vi "多参数数据插入.vi"(8 "error in (no error)":errorcluster caption="错误输入（无错误）", 9 "编号":string, 10 "columns enable":T1, 11 "data in":T2) -> (0 "error out":errorcluster)   [LabVIEW 2016, in "斯坦道多参数.lvlib"]
uses:
  <vilib>/Utility/sysdir.llb/System Directory Type.ctl
  <vilib>/addons/database/Auxilliary.llb/DB Tools Parameter Info.ctl
  <vilib>/addons/database/Auxilliary.llb/DB Tools DataTypes.ctl
  <vilib>/addons/database/Auxilliary.llb/DB Tools Parameter Dir.ctl
  <vilib>/addons/database/Auxilliary.llb/DB Tools Column Info.ctl
  <vilib>/addons/database/Auxilliary.llb/DB Tools Format Datetime String (Time Stamp).vi
  <vilib>/addons/database/Connection.llb/DB Tools Open Connec (String).vi
  <vilib>/addons/database/Connection.llb/Conn Execute.vi
  <vilib>/addons/database/Recordset.llb/Rec Destroy - Connection.vi
  <vilib>/addons/database/Command.llb/Cmd Set Parameter Value (C).vi
  <vilib>/addons/database/Command.llb/Cmd Execute.vi
  <vilib>/addons/database/Recordset.llb/Rec Destroy - Command.vi
  <vilib>/addons/database/Command.llb/Cmd Delete.vi
  <vilib>/addons/database/NI_Database_API.lvlib
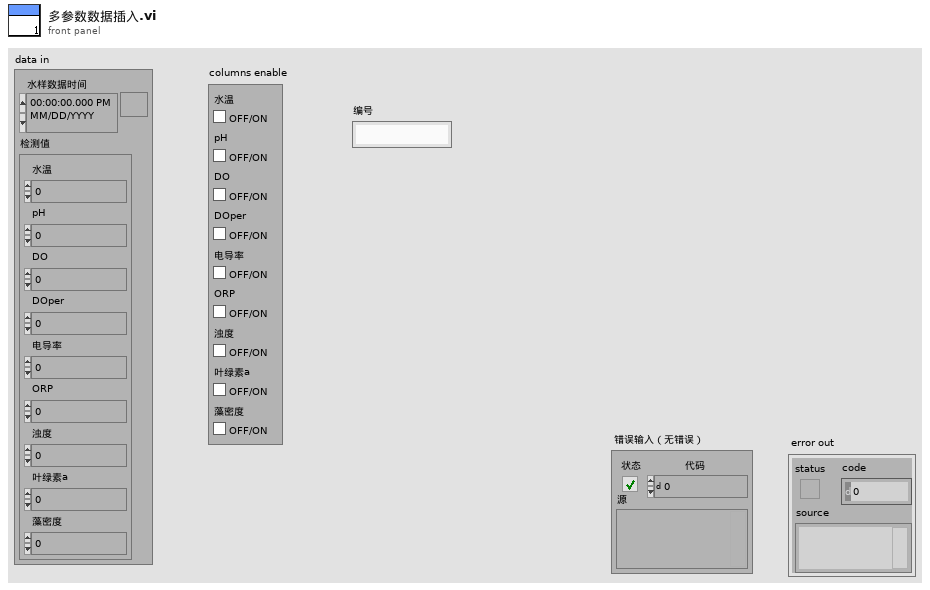
[diagram p1: front panel]
types:
  T1 = cluster{"水温":bool, "pH":bool, "DO":bool, "DOper":bool, "电导率":bool, "ORP":bool, "浊度":bool, "叶绿素a":bool, "藻密度":bool}
  T2 = cluster{"水样数据时间":timestamp, "检测值":cluster{"水温":dbl, "pH":dbl, "DO":dbl, "DOper":dbl, "电导率":dbl, "ORP":dbl, "浊度":dbl, "叶绿素a":dbl, "藻密度":dbl}}
  T3 = typedef "System Directory Type.ctl" = i32
  T4 = cluster{"水温":dbl, "pH":dbl, "DO":dbl, "DOper":dbl, "电导率":dbl, "ORP":dbl, "浊度":dbl, "叶绿素a":dbl, "藻密度":dbl}
  T5 = typedef "NI_Database_API.lvlib/DB Tools Column Info.ctl" = cluster{"column name":string, "data type":T6, "size":i32, "allow null?":bool}
  T6 = typedef "NI_Database_API.lvlib/DB Tools DataTypes.ctl" = enum16{"String", "Long (I32)", "Single (SGL)", "Double (DBL)", "Date/Time", "Binary"}
  T7 = typedef "NI_Database_API.lvlib/DB Tools Parameter Info.ctl" = cluster{"parameter name":string, "type":T6, "direction":T8, "value":variant}
  T8 = typedef "NI_Database_API.lvlib/DB Tools Parameter Dir.ctl" = enum32{"Input", "Output", "Input/Output", "Return Value"}
  T9 = typedef "NI_Database_API.lvlib/Conn ObjectReference.ctl" = refnum<k1>
  T10 = typedef "NI_Database_API.lvlib/Rec ObjectReference.ctl" = refnum<k1>
  T11 = typedef "NI_Database_API.lvlib/Cmd ObjectReference.ctl" = refnum<k1>
  T12 = typedef "NI_Database_API.lvlib/Cmd-Rec Object Reference.ctl" = refnum<k1>
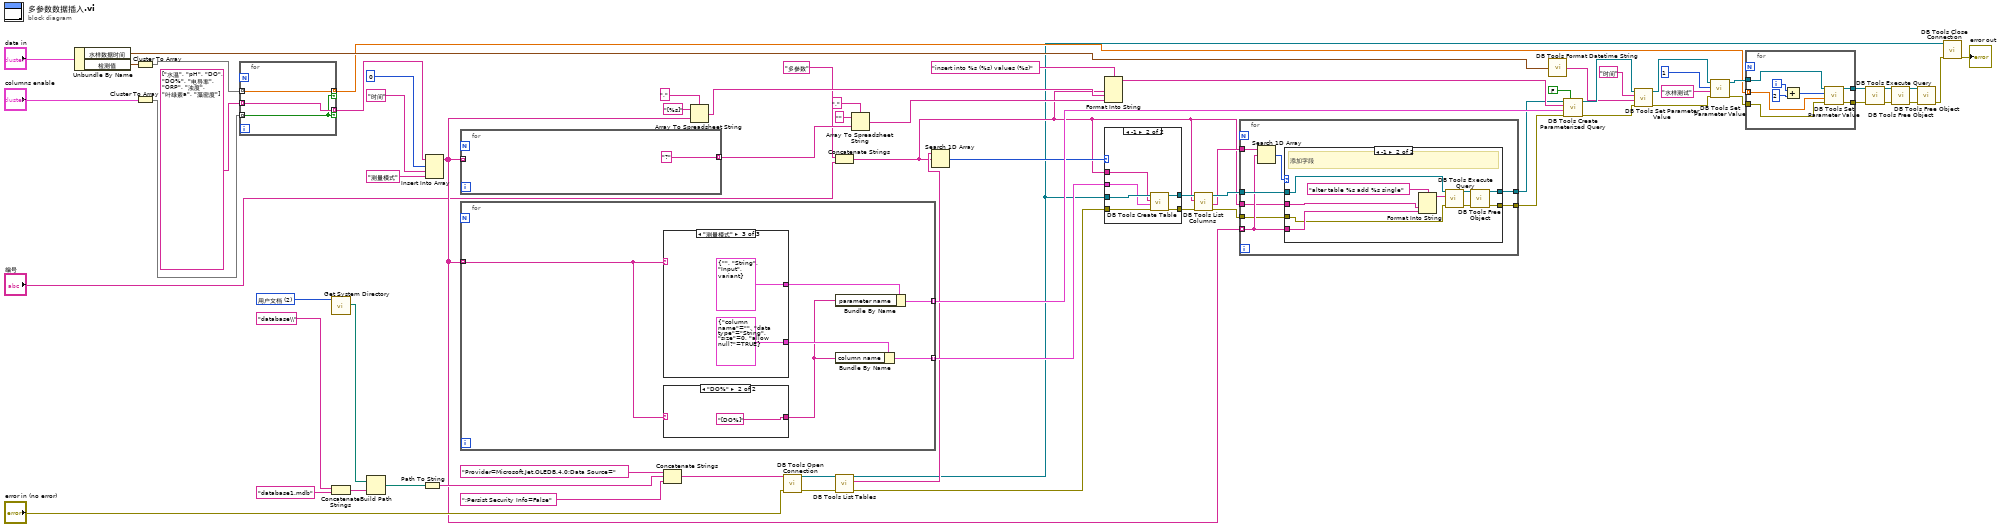
[diagram p0: block diagram]
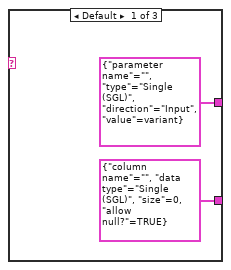
[diagram p5: hidden frame]
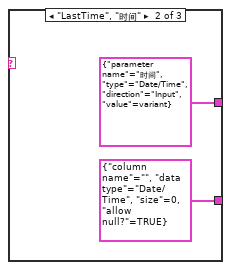
[diagram p6: hidden frame]
diagram:
  w70 = T3 2 items=["用户目录"=0, "用户桌面"=1, "用户文档"=2, "用户应用程序数据"=3, "用户设置"=4, "用户临时目录"=5, "公共文档"=6, "公共应用程序数据"=7, "公共设置"=8, "公共缓存"=13, "系统核心库"=9, "系统安装库"=10, "应用程序文件"=11, "启动盘根目录"=12] ("system directory type")
  n1 = Unbundle By Name("data in") -> ("水样数据时间"=w29:timestamp, "检测值"=w19:T4)
  n2 = Cluster To Array(cluster=w19) -> (array=w18:dbl[])
  n3 = Cluster To Array(cluster="columns enable") -> (array=w55:bool[])
  n4 = for {
    tunnel: string[] ["水温", "pH", "DO", "DO%", "电导率", "ORP", "浊度", "叶绿素a", "藻密度"] ("columns name") -> [w73] mode=indexing
    tunnel: w55 -> [w71] mode=indexing
    tunnel: [w73] -> w6 mode=indexing if=w71
    tunnel: w18 -> [w72] mode=indexing
    tunnel: [w72] -> w17 mode=indexing if=w71
  }
  n5 = call <vilib>:"Get System Directory.vi"("system directory type"=w70) -> ("system directory"=w68:path)  [unwired: 10 in]
  n6 = Concatenate Strings("database\\" ("condition"), "database1.mdb" ("字符串")) -> (w62:string)
  n7 = Build Path(base path=w68, name or relative path=w62) -> (appended path=w67:path)
  n8 = Path To String(path=w67) -> (string=w66:string)
  n9 = Insert Into Array(array=w6, index=0 ("索引"), new element #1="时间" ("新元素/子数组"), new element #2="测量模式" ("新元素/子数组")) -> (w14:string[])
  n10 = for {
    tunnel: w14 -> [_] mode=indexing
    tunnel: ["?"] -> w42 mode=indexing
  }
  n11 = for {
    tunnel: w14 -> [w76] mode=indexing
    tunnel: [w77] -> w41 mode=indexing
    tunnel: [w79] -> w40 mode=indexing
    n12 = case shown="\"测量模式\"" w76 {
      tunnel: [T7 {"parameter name"="", "type"=enum."Single (SGL)", "direction"=enum."Input", "value"=variant} ("parameter information") T7 {"parameter name"="时间", "type"=enum."Date/Time", "direction"=enum."Input", "value"=variant} ("parameter information") T7 {"parameter name"="", "type"=enum."String", "direction"=enum."Input", "value"=variant} ("parameter information")] -> w78
      tunnel: [T5 {"column name"="", "data type"=enum."Single (SGL)", "size"=0, "allow null?"=TRUE} ("column information") T5 {"column name"="", "data type"=enum."Date/Time", "size"=0, "allow null?"=TRUE} ("column information") T5 {"column name"="", "data type"=enum."String", "size"=0, "allow null?"=TRUE} ("column information")] -> w80
      frame Default {
      }
      frame "LastTime", "时间" {
      }
      frame "测量模式" {
      }
    }
    n13 = case shown="\"DO%\"" w76 {
      selector: w76 -> [w81 _]
      tunnel: [w81 "[DO%]"] -> w75
      frame "假", Default {
      }
      frame "DO%" {
      }
    }
    n14 = Bundle By Name(cluster=w78, "parameter name"=w75) -> (w77:T7)
    n15 = Bundle By Name(cluster=w80, "column name"=w75) -> (w79:T5)
  }
  n16 = Concatenate Strings("Provider=Microsoft.Jet.OLEDB.4.0;Data Source=" ("condition"), w66, ";Persist Security Info=False" ("condition")) -> (w64:string)
  n17 = Array To Spreadsheet String(delimiter (Tab)="," ("分隔符(Tab)"), array=w14, 3:"[%s]" ("格式字符串")) -> (spreadsheet string=w51:string)
  n18 = call-poly <vilib>:"DB Tools Open Connection.vi"("error in (no error)"="error in (no error)", "connection information"=w64) -> ("error out"=w59:errorcluster, "connection reference"=w2:T9)  [unwired: 6 in]
  n19 = Concatenate Strings("多参数" ("字符串"), "编号") -> (w3:string)
  n20 = call <vilib>:"DB Tools List Tables.vi"("error in (no error)"=w59, "connection reference"=w2) -> ("error out"=w39:errorcluster, "tables"=w37:string[], "connection reference out"=w1:T9)  [unwired: 3 in]
  n21 = Array To Spreadsheet String(delimiter (Tab)="," ("分隔符(Tab)"), array=w42, 3:"" ("格式字符串")) -> (spreadsheet string=w46:string)
  n22 = Search 1D Array(1D array=w37, element=w3) -> (index of element=w36:i32)  [unwired: 1 in]
  n23 = Format Into String(format string="insert into %s (%s) values (%s)" ("格式字符串"), w3, w51, w46) -> (resulting string=w45:string)  [unwired: 2 in, 1 out]
  n24 = case shown="-1" w36 {
    tunnel: w1 -> [w90 w96]
    tunnel: [w90 w95] -> w13
    tunnel: [w89 w94] -> w11
    tunnel: w40 -> [_ w92]
    tunnel: w39 -> [w89 w93]
    tunnel: w3 -> [_ w91]
    frame 0, Default {
    }
    frame -1 {
      n25 = call <vilib>:"DB Tools Create Table.vi"("error in (no error)"=w93, "column information"=w92, "table"=w91, "connection reference"=w96) -> ("error out"=w94:errorcluster, "connection reference out"=w95:T9)  [unwired: 4 in]
    }
  }
  n26 = call <vilib>:"DB Tools List Columns.vi"("error in (no error)"=w11, "table"=w3, "connection reference"=w13) -> ("error out"=w9:errorcluster, "columns"=w10:string[], "connection reference out"=w12:T9)  [unwired: 1 in, 1 out]
  n27 = for {
    tunnel: w14 -> [w101] mode=indexing
    tunnel: w12 -> [w102]
    tunnel: w10 -> [w104]
    tunnel: w9 -> [w100]
    tunnel: [w99] -> w7
    tunnel: [w98] -> w8
    tunnel: w3 -> [w97]
    n28 = Search 1D Array(1D array=w104, element=w101) -> (index of element=w103:i32)  [unwired: 1 in]
    n29 = case shown="-1" w103 {
      tunnel: [w106 w112] -> w98
      tunnel: [w105 w111] -> w99
      tunnel: w102 -> [w106 w110]
      tunnel: w101 -> [_ w109]
      tunnel: w100 -> [w105 w108]
      tunnel: w97 -> [_ w107]
      frame 0, Default {
      }
      frame -1 {
        # "添加字段"
        n30 = Format Into String(format string="alter table %s add %s single", w107, w109) -> (resulting string=w113:string)  [unwired: 2 in, 1 out]
        n31 = call-poly <vilib>:"DB Tools Execute Query.vi"("error in (no error)"=w108, "SQL query"=w113, "connection reference"=w110) -> ("error out"=w115:errorcluster, "recordset reference"=w116:T10)  [unwired: 5 in]
        n32 = call-poly <vilib>:"DB Tools Free Object.vi"("error in (no error)"=w115, "recordset reference"=w116) -> ("error out"=w111:errorcluster, "connection reference"=w112:T9)  [unwired: 8 in]
      }
    }
  }
  n33 = call-poly <vilib>:"DB Tools Format Datetime String.vi"("time stamp"=w29) -> ("date/time string"=w28:string)
  n34 = call <vilib>:"DB Tools Create Parameterized Query.vi"("auto-detect parameters? (F)"=FALSE, "error in (no error)"=w7, "parameters"=w41, "SQL query"=w45, "connection reference"=w8) -> ("error out"=w44:errorcluster, "command reference"=w43:T11)  [unwired: 2 in, 1 out]
  n35 = call-poly <vilib>:"DB Tools Set Parameter Value.vi"("error in (no error)"=w44, "value"=w28, "parameter index"="时间", "command reference"=w43) -> ("error out"=w25:errorcluster, "command reference out"=w26:T11)  [unwired: 4 in]
  n36 = call-poly <vilib>:"DB Tools Set Parameter Value.vi"("error in (no error)"=w25, "value"="水样测试", "parameter index"=1, "command reference"=w26) -> ("error out"=w20:errorcluster, "command reference out"=w21:T11)  [unwired: 4 in]
  n37 = for {
    tunnel: w21 -> [w120]
    tunnel: w20 -> [w121]
    tunnel: w17 -> [w119] mode=indexing
    tunnel: [w118] -> w16
    tunnel: [w117] -> w15
    i -> [w124]
    n38 = Add(x=w124, y=2) -> (x+y=w122:i32)
    n39 = call-poly <vilib>:"DB Tools Set Parameter Value.vi"("error in (no error)"=w121, "value"=w119, "parameter index"=w122, "command reference"=w120) -> ("error out"=w117:errorcluster, "command reference out"=w118:T11)  [unwired: 4 in]
  }
  n40 = call-poly <vilib>:"DB Tools Execute Query.vi"("error in (no error)"=w15, "command reference"=w16) -> ("error out"=w33:errorcluster, "command-recordset reference"=w34:T12)  [unwired: 6 in]
  n41 = call-poly <vilib>:"DB Tools Free Object.vi"("error in (no error)"=w33, "command-recordset reference"=w34) -> ("error out"=w32:errorcluster, "command reference"=w31:T11)  [unwired: 8 in]
  n42 = call-poly <vilib>:"DB Tools Free Object.vi"("error in (no error)"=w32, "command reference"=w31) -> ("error out"=w30:errorcluster)  [unwired: 8 in, 1 out]
  n43 = call <vilib>:"DB Tools Close Connection.vi"("error in (no error)"=w30, "connection reference"=w1) -> ("error out"=→"error out":errorcluster)  [unwired: 5 in]
